vi "Edgertronic-image2.vi"(3 "error in (no error)":errorcluster, 5 "URL":string="192.168.1.101") -> (0 "error out":errorcluster, 1 "Image:":T1={"Connection Information:"="", "URL redirect to JPEG image"="20140911165611"}, 2 "new picture":picture)   [LabVIEW 2015]
doc: "This VI returns a URL redirect to the actual JPEG image."
panel:
  in  "Zoom Factor":sgl=0.5
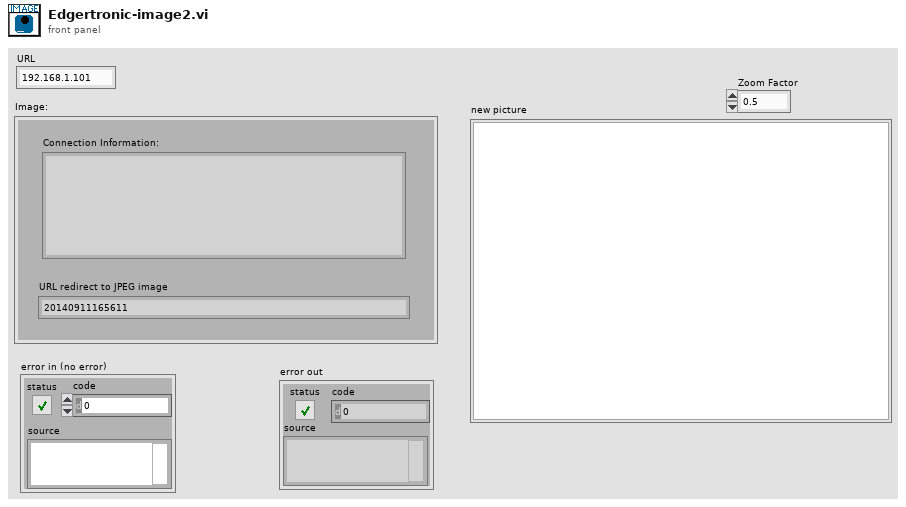
[diagram p1: front panel]
types:
  T1 = cluster{"Connection Information:":string, "URL redirect to JPEG image":string}
  T2 = enum16{"big-endian, network order", "native, host order", "little-endian"}
  T3 = typedef "imagedata.ctl" = cluster{"image type":i32, "image depth":i32, "image":u8[], "mask":u8[], "colors":u32[], "Rectangle":cluster{"left":i16, "top":i16, "right":i16, "bottom":i16}}
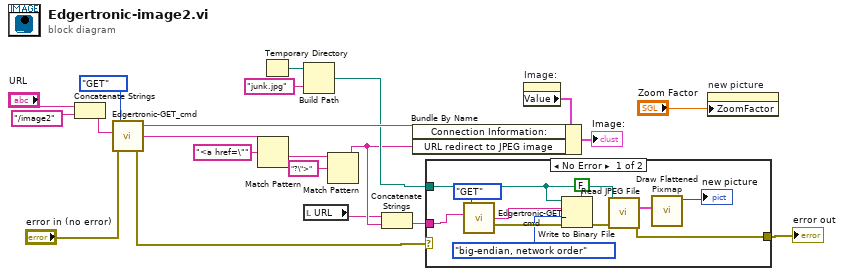
[diagram p0: block diagram]
diagram:
  n1 = Concatenate Strings("URL", "/image2" ("GET Cmd")) -> (w5:string)
  n2 = call "Edgertronic-GET_cmd.vi"("error in (no error)"="error in (no error)", "URL"=w5, "Type"=enum16{"GET", "POST"}."GET") -> ("error out"=w14:errorcluster, "data"=w15:string, "Connection Info"=w16:string)  [unwired: 1 in]
  n3 = Match Pattern(string=w15, regular expression="<a href=\"") -> (after substring=w19:string)  [unwired: 1 in, 3 out]
  n4 = Temporary Directory() -> (w10:path)
  n5 = Build Path(base path=w10, name or relative path="junk.jpg") -> (appended path=w9:path)
  n6 = local read "URL"() -> (w1:string)
  n7 = Match Pattern(string=w19, regular expression="?\">") -> (before substring=w4:string)  [unwired: 1 in, 3 out]
  n8 = Concatenate Strings(w1, w4) -> (w2:string)
  n9 = case shown="No Error" w14 {
    selector: w14 -> [_ w33]
    tunnel: w2 -> [w23 _]
    tunnel: [w29 w33] -> w13
    tunnel: w9 -> [w28 _]
    frame No Error {
      n10 = call "Edgertronic-GET_cmd.vi"("URL"=w23, "Type"=enum16{"GET", "POST"}."GET") -> ("error out"=w30:errorcluster, "data"=w25:string)  [unwired: 2 in, 1 out]
      n11 = Write to Binary File(file (use dialog)=w28, data=w25, error in=w30, 5:FALSE ("prepend array or string size? (T)"), 9:T2."big-endian, network order" ("byte order (0:big-endian, network order)")) -> (error out=w32:errorcluster)  [unwired: 1 in, 2 out]
      n12 = call <vilib>:"Read JPEG File.vi"("error in (no error)"=w32, "path to JPEG file"=w28) -> ("error out"=w29:errorcluster, "image data"=w31:T3)  [unwired: 7 in, 1 out]
      n13 = call <vilib>:"Draw Flattened Pixmap.vi"("image data"=w31) -> ("new picture"=→"new picture":picture)  [unwired: 8 in]
    }
    frame Error {
    }
  }
  "error out" <- w13
  n14 = property on="Image:" class="Clust (strict)"() -> ("Value"=w17:T1)  [unwired: 2 in, 2 out]
  n15 = Bundle By Name(cluster=w17, "Connection Information:"=w16, "URL redirect to JPEG image"=w4) -> (→"Image:":T1)
  n16 = property on="new picture" class="Pict"("ZoomFactor"="Zoom Factor") -> ()  [unwired: 2 in, 2 out]
